vi "Fpga-Hardware-Exerciser.vi"() -> ()   [LabVIEW 2017]
uses:
  <vilib>/Platform/TimedLoop/XDataNode/XDataNode.xnode
  <vilib>/Platform/TimedLoop/XDataNode/nitl_modes.ctl
  <vilib>/Platform/TimedLoop/XDataNode/XDNodeRunTimeDep.lvlib
  <vilib>/Platform/TimedLoop/XDataNode/wakeup.ctl
  <vilib>/Platform/TimedLoop/XDataNode/timing_clust.ctl
  <vilib>/rvi/DataTransferAndStorage/Container/XNode/niFpgaContainer.xnode
  <vilib>/rvi/interface/RandomDataEmulation/nirviRandomDataFpgaReadWriteTemplate.vi
  <vilib>/rvi/IPIntegrationNode/IPINode_Xnode/niFpgaIPINode.xnode
  IP_Block_1SimFiles/xsim.dir/d_microblaze_wrapper_top/xsimkD566ABB023B84B7CB0097135CB091ED7.dll
  <vilib>/rvi/IPIntegrationNode/IPINode_Typedef/niFpgaIPINodeSupportedFamilies.ctl
  <vilib>/rvi/IPIntegrationNode/IPINode_Utilities/niFpgaIPINodeSimCore.vi
panel:
  out "tdata_LastNonZero":u32
  out "tlast_Count":u16
  out "tvalid_Count":u16
  out "AXI_STR_RXD_tready_Count":u16
  out "tlast":bool
  out "tdata":u32
  out "tvalid":bool
  in  "sys_reset":bool
  out "AXI_STR_RXD_tready":bool
  out "GPIO2_tri_o":u32 format="%.0x"
  in  "GPIO1_tri_i":u32
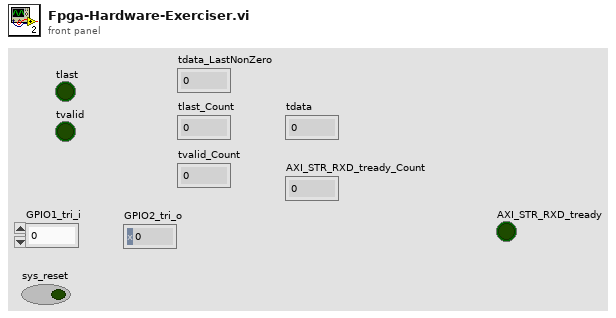
[diagram p1: front panel]
types:
  T1 = typedef "XDNodeRunTimeDep.lvlib/timing_clust.ctl" = cluster{"Expected End [f-1]":u64, "Actual End [f-1]":u64, "Finished Late? [f-1]":bool, "Expected End [i-1]":u64, "Actual End [i-1]":u64, "Finished Late? [i-1]":bool, "Expected Start [i]":u64, "Actual Start [i]":u64, "Expected Start [f]":u64, "Actual Start [f]":u64, "Source Name":string, "Structure Name":string, "Period":i64, "Deadline":i64, "Offset":i64, "Start":i64, "Priority":i32, "Timeout":i32, "Mode":T2, "Wakeup Reason":T3, "Error":errorcluster, "Source Type":string, "Secondary Source Type":string, "Global End Time":u64, "Global Start Time":u64, "Frame Duration":u64, "Iteration Duration":u64, "Assigned CPU":i32, "I/O Scan Engine Mode":u32}
  T2 = typedef "XDNodeRunTimeDep.lvlib/nitl_modes.ctl" = enum32{"No Change", "Process missed periods, maintain original phase", "Discard missed periods, maintain original phase", "Process missed periods, ignore original phase", "Discard missed periods, ignore original phase"}
  T3 = typedef "XDNodeRunTimeDep.lvlib/wakeup.ctl" = enum32{"Normal", "Aborted", "Asynchronous wakeup", "Timing source error", "Timed loop error", "Timeout"}
  T4 = typedef "niFpgaIPINodeSupportedFamilies.ctl" = cluster{"unlimited?":bool, "supported targets":string[]}
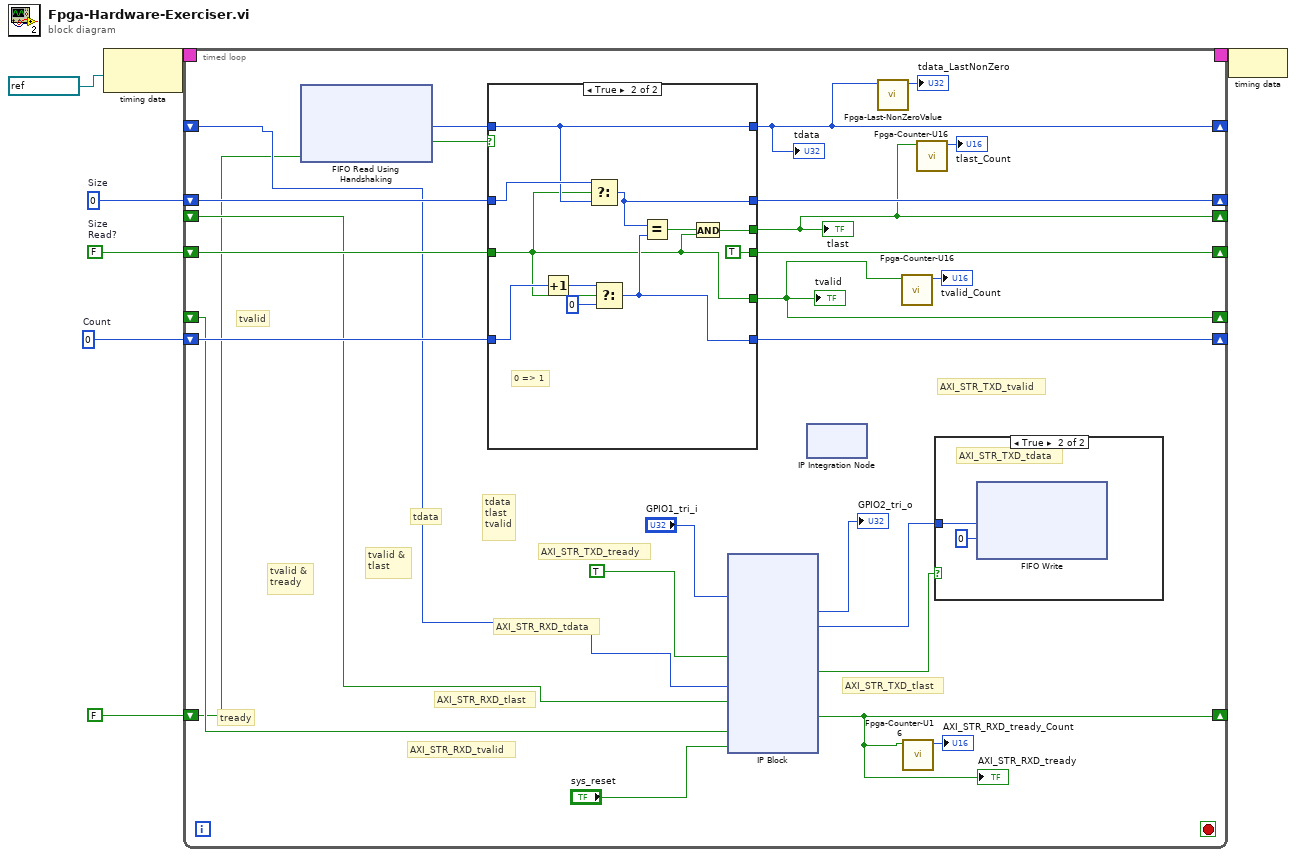
[diagram p0: block diagram]
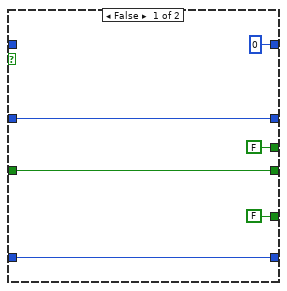
[diagram p3: hidden frame]
diagram:
  w2 = u32 0  # Count
  w4 = FALSE  # Size Read?
  w3 = u32 0  # Size
  n1 = node-c288(refnum<k21> "100MHz" ("Source Name")) -> (w7:T1)
  n2 = timed-loop {
    timing: w7 -> [_]
    timing-out: [_] -> w6
    shift-right: [w31] -> _
    shift-left: w4 -> [w32]
    shift-right: [w28] -> _
    shift-left: w3 -> [w30]
    shift-right: [w22] -> _
    shift-left: w2 -> [w23]
    shift-right: [w13] -> _
    shift-left: _ -> [w21]
    shift-right: [w15] -> _
    shift-left: FALSE ("AXI_STR_RXD_tready") -> [w18]
    shift-right: [w9] -> _
    shift-left: _ -> [w19]
    shift-right: [w11] -> _
    shift-left: _ -> [w20]
    stop <- _ stop-if-true
    # "AXI_STR_TXD_tlast"
    # "AXI_STR_TXD_tvalid"
    # "AXI_STR_TXD_tready"
    # "AXI_STR_RXD_tvalid"
    # "AXI_STR_RXD_tlast"
    # "AXI_STR_RXD_tdata"
    # "tdata"
    # "tvalid &\ntlast"
    # "tvalid"
    # "tready"
    # "tvalid &\ntready"
    # "tdata\ntlast\ntvalid"
    n3 = xnode ("FIFO Read Using Handshaking")("Ready for Output"=w18) -> ("Element"=w29:u32, "Output Valid"=w33:bool)  [unwired: 1 in, 1 out]
    n4 = case shown="True" w33 {
      tunnel: w32 -> [w124 w126]
      tunnel: [w124 TRUE ("Size\nRead?")] -> w31
      tunnel: w30 -> [w125 w136]
      tunnel: w29 -> [_ w131]
      tunnel: [w125 w130] -> w28
      tunnel: w23 -> [w123 w135]
      tunnel: [w123 w129] -> w22
      tunnel: [FALSE ("Size\nRead?") w126] -> w13
      tunnel: [u32 0 ("Element") w131] -> w9
      tunnel: [FALSE w127] -> w11
      frame False {
      }
      frame True {
        # "0 => 1"
        n5 = Increment(x=w135) -> (x+1=w133:u32)
        n6 = Select(t=w136, s=w126, f=w131) -> (s? t:f=w130:u32)
        n7 = Select(t=w133, s=w126, f=u32 0) -> (s? t:f=w129:u32)
        n8 = Equal?(x=w130, y=w129) -> (x = y?=w128:bool)
        n9 = And(x=w128, y=w126) -> (x .and. y?=w127:bool)
      }
    }
    "tvalid" <- w13
    "tdata" <- w9
    "tlast" <- w11
    n10 = xnode ("IP Block")("GPIO1_tri_i"="GPIO1_tri_i", "AXI_STR_TXD_tready"=TRUE, "AXI_STR_RXD_tdata"=w19, "AXI_STR_RXD_tlast"=w20, "AXI_STR_RXD_tvalid"=w21, "sys_reset"="sys_reset") -> ("GPIO2_tri_o"=→"GPIO2_tri_o":u32, "AXI_STR_TXD_tdata"=w17:u32, "AXI_STR_TXD_tvalid"=w16:bool, "AXI_STR_RXD_tready"=w15:bool)  [unwired: 2 out]
    "AXI_STR_RXD_tready" <- w15
    n11 = xnode "IP Integration Node"() -> ()
    n12 = call "Fpga-Last-NonZeroValue.vi"("d_mcs_i\\IO_BUS_write_data in"=w9) -> ("d_mcs_i\\IO_BUS_write_data out"=→"tdata_LastNonZero":u32)  [unwired: 10 in]
    n13 = call "Fpga-Counter-U16.vi"("d_mcs_i\\IO_BUS_read_strobe"=w13) -> ("Numeric"=→"tvalid_Count":u16)  [unwired: 10 in]
    n14 = call "Fpga-Counter-U16.vi"("d_mcs_i\\IO_BUS_read_strobe"=w15) -> ("Numeric"=→"AXI_STR_RXD_tready_Count":u16)  [unwired: 10 in]
    n15 = call "Fpga-Counter-U16.vi"("d_mcs_i\\IO_BUS_read_strobe"=w11) -> ("Numeric"=→"tlast_Count":u16)  [unwired: 10 in]
    n16 = case shown="True" w16 {
      tunnel: w17 -> [_ w119]
      frame False {
      }
      frame True {
        # "AXI_STR_TXD_tdata"
        n17 = xnode ("FIFO Write")("Element"=w119, "Timeout"=0) -> ()  [unwired: 1 in, 2 out]
      }
    }
  }
  n18 = node-c288(w6) -> ()
